vi "SVFA Compensate Phase for Time Delay (NxM).vi"(0 "phase spectra":cluster{"f0":dbl, "df":dbl, "phase":dbl[]}[][](array[cluster]) {"phase" format="%.2f"; "df" format="%.2f"; "f0" format="%.2f"}, 2 "delays [s]":dbl[][](array[numeric]) format="%#_4p", 4 "spectrum info":T1[][](array[typedef]) {"x-axis units" items=["Time (s)"=0, "Frequency-CB (Hz)"=1, "Frequency-CPB (Hz)"=1248, "Frequency-Arbitrary (Hz)"=2357, "Quefrency (s)"=2, "Revolutions (rev)"=3, "Order"=4, "Speed (RPM)"=11, "Speed (rad/s)"=21, "Index"=65535]; "weighting filter" items=["Linear", "A-weighting", "B-weighting", "C-weighting", "ITU-R 468-4", "Dolby", "CCITT", "C-message", "Wb", "Wc", "Wd", "We", "Wf", "Wh", "Wj", "Wk", "Wm", "AES17 20 kHz lowpass", "AES17 40 kHz lowpass", "AES17 20 kHz highpass", "AES17 40 kHz highpass"]; "dB reference [EU]" format="%.2f"; "engineering units" items=["custom..."=0, "V"=1, "A"=21, "C"=30, "pC"=31, "s"=32, "-"=29, "Pa"=2, "N"=20, "g"=3, "m/s^2"=4, "m/s"=5, "m"=6, "mm/s"=12, "mm"=13, "micron/s"=14, "micron"=15, "in/s^2"=7, "in/s"=8, "in"=9, "mil/s"=10, "mil"=11, "rad/s^2"=16, "rad/s"=17, "rad"=18, "deg/s^2"=26, "deg/s"=27, "deg"=28, "RPM"=22, "cycle/s^2"=23, "Hz"=24, "cycle"=25, "strain"=19]; "spectral info"."window" items=["None "=0, "Hanning"=1, "Hamming"=2, "Blackman-Harris"=3, "Exact Blackman"=4, "Blackman"=5, "Flat Top"=6, "4 Term B-Harris "=7, "7 Term B-Harris"=8, "Low Sidelobe"=9, "Force - Exponential"=10, "Gaussian"=62]}, 5 "error in (no error)":errorcluster) -> (14 "compensated phase spectra":cluster{"f0":dbl, "df":dbl, "phase":dbl[]}[][](array[cluster]) {"phase" format="%.2f"; "df" format="%.2f"; "f0" format="%.2f"}, 15 "unit labels":string[][](array[string]), 18 "dup spectrum info":T1[][](array[typedef]) {"x-axis units" items=["Time (s)"=0, "Frequency-CB (Hz)"=1, "Frequency-CPB (Hz)"=1248, "Frequency-Arbitrary (Hz)"=2357, "Quefrency (s)"=2, "Revolutions (rev)"=3, "Order"=4, "Speed (RPM)"=11, "Speed (rad/s)"=21, "Index"=65535]; "weighting filter" items=["Linear", "A-weighting", "B-weighting", "C-weighting", "ITU-R 468-4", "Dolby", "CCITT", "C-message", "Wb", "Wc", "Wd", "We", "Wf", "Wh", "Wj", "Wk", "Wm", "AES17 20 kHz lowpass", "AES17 40 kHz lowpass", "AES17 20 kHz highpass", "AES17 40 kHz highpass"]; "dB reference [EU]" format="%.2f"; "engineering units" items=["custom..."=0, "V"=1, "A"=21, "C"=30, "pC"=31, "s"=32, "-"=29, "Pa"=2, "N"=20, "g"=3, "m/s^2"=4, "m/s"=5, "m"=6, "mm/s"=12, "mm"=13, "micron/s"=14, "micron"=15, "in/s^2"=7, "in/s"=8, "in"=9, "mil/s"=10, "mil"=11, "rad/s^2"=16, "rad/s"=17, "rad"=18, "deg/s^2"=26, "deg/s"=27, "deg"=28, "RPM"=22, "cycle/s^2"=23, "Hz"=24, "cycle"=25, "strain"=19]; "spectral info"."window" items=["None "=0, "Hanning"=1, "Hamming"=2, "Blackman-Harris"=3, "Exact Blackman"=4, "Blackman"=5, "Flat Top"=6, "4 Term B-Harris "=7, "7 Term B-Harris"=8, "Low Sidelobe"=9, "Force - Exponential"=10, "Gaussian"=62]}, 19 "error out":errorcluster)   [LabVIEW 2017]
doc: "Compensates FFT and frequency response phase spectra for time delay. You can introduce time delays with the DUT, data acquisition hardware, and measurement analysis. Compensation in this VI is restricted to linear phase resulting from a pure time delay. Wire data to the <B>phase spectrum</B> input to determine the polymorphic instance to use or manually select the instance."
uses:
  <vilib>/addons/_NISVFA/_Shared subVIs/Controls/svc_Spectrum Info.ctl
  <vilib>/addons/_NISVFA/_Shared subVIs/Controls/svc_X-Axis Units.ctl
  <vilib>/addons/_NISVFA/_Shared subVIs/Controls/svc_Spectrum Type.ctl
  <vilib>/addons/_NISVFA/_Shared subVIs/Controls/svc_Engineering Units Text Ring.ctl
  <vilib>/addons/_NISVFA/_Shared subVIs/Controls/svc_Weighting Filter Text Ring.ctl
  <vilib>/addons/_NISVFA/_Shared subVIs/Controls/svc_Complimentary Spectrum Units.ctl
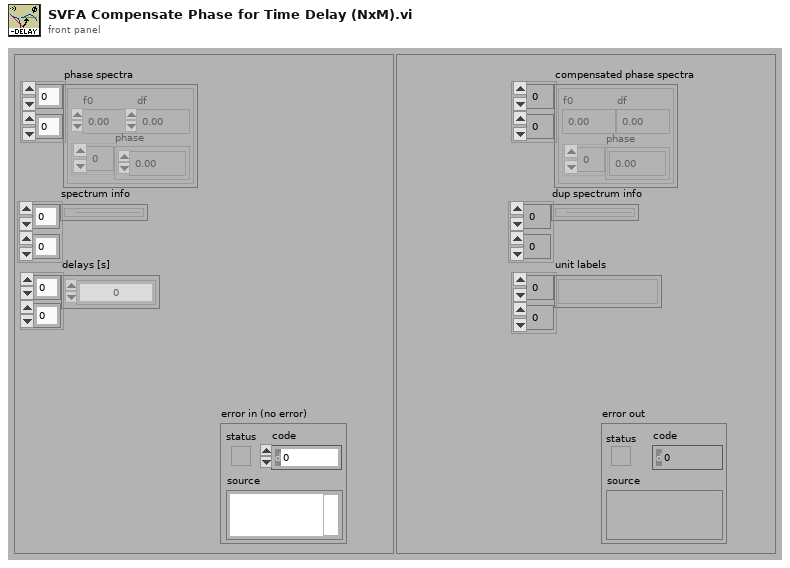
[diagram p1: front panel]
types:
  T1 = typedef "svc_Spectrum Info.ctl" = cluster{"channel name":string, "description":string, "x-axis units":T2, "spectral info":cluster{"spectrum type":T3, "linear/dB":enum16{"linear", "dB"}, "window":u16, "window size":i32, "FFT size":i32}, "engineering units":T4, "custom label":string, "dB reference [EU]":dbl, "peak units":enum16{"rms", "peak", "peak-peak"}, "weighting filter":T5, "spectral density?":bool, "unit label":string, "spectrum skewed?":bool, "complimentary spectrum units":T6}
  T2 = typedef "svc_X-Axis Units.ctl" = u16
  T3 = typedef "svc_Spectrum Type.ctl" = enum16{"FFT Spectrum [complex]", "Amplitude [Magnitude]", "Power [Magnitude^2]", "Cross Spectrum [complex]", "Frequency Response [Complex]"}
  T4 = typedef "svc_Engineering Units Text Ring.ctl" = u16
  T5 = typedef "svc_Weighting Filter Text Ring.ctl" = u16
  T6 = typedef "svc_Complimentary Spectrum Units.ctl" = enum16{"none", "radians", "degrees", "cycles", "imaginary"}
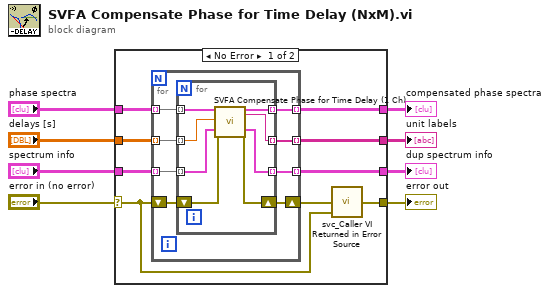
[diagram p0: block diagram]
diagram:
  n1 = case shown="No Error" "error in (no error)" {
    selector: "error in (no error)" -> [w14 w35]
    tunnel: "phase spectra" -> [w16 w36]
    tunnel: [w15 w36] -> w7
    tunnel: [w17 w35] -> w5
    tunnel: "delays [s]" -> [w10 _]
    tunnel: "spectrum info" -> [w12 w34]
    tunnel: [w11 w34] -> w2
    tunnel: [w9 _] -> w1
    frame No Error {
      n2 = for {
        tunnel: w16 -> [w25] mode=indexing
        tunnel: [w24] -> w15 mode=indexing
        shift-right: [w22] -> w13
        shift-left: w14 -> [w23]
        tunnel: w12 -> [w21] mode=indexing
        tunnel: [w20] -> w11 mode=indexing
        tunnel: w10 -> [w18] mode=indexing
        tunnel: [w19] -> w9 mode=indexing
        n3 = for {
          tunnel: w25 -> [w33] mode=indexing
          tunnel: [w32] -> w24 mode=indexing
          tunnel: w21 -> [w29] mode=indexing
          tunnel: [w28] -> w20 mode=indexing
          tunnel: [w27] -> w19 mode=indexing
          tunnel: w18 -> [w26] mode=indexing
          shift-right: [w30] -> w22
          shift-left: w23 -> [w31]
          n4 = call <vilib>:"SVFA Compensate Phase for Time Delay (1 Ch).vi"("phase spectrum"=w33, "delay [s]"=w26, "spectrum info"=w29, "error in (no error)"=w31) -> ("compensated phase spectrum"=w32:cluster{"f0":dbl, "df":dbl, "phase":dbl[]}, "unit label"=w27:string, "dup spectrum info"=w28:T1, "error out"=w30:errorcluster)  [unwired: 12 in]
        }
      }
      n5 = call <vilib>:"svc_Caller VI Returned in Error Source.vi"("warning input to caller"=w14, "error in (no error)"=w13) -> ("error out"=w17:errorcluster)  [unwired: 3 in]
    }
    frame Error {
    }
  }
  "compensated phase spectra" <- w7
  "error out" <- w5
  "dup spectrum info" <- w2
  "unit labels" <- w1
